vi "Refresh Item.vi"(8 "error in (no error)":errorcluster, 10 "Item Index":i32, 11 "BetterBoxHandle in":refnum<class "BetterBoxHandle.lvclass">) -> (0 "error out":errorcluster, 3 "BetterBoxHandle out":refnum<class "BetterBoxHandle.lvclass">)   [LabVIEW 2020, in "BetterDragAndDrop.lvlib" / "BetterBoxHandle.lvclass"]
uses:
  BetterBoxHandle.lvclass
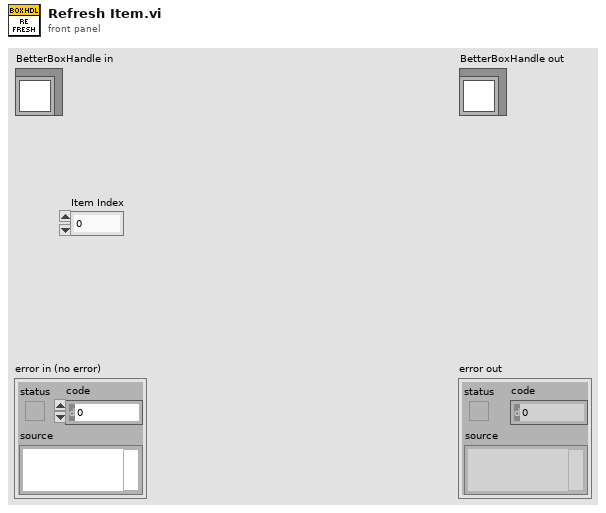
[diagram p1: front panel]
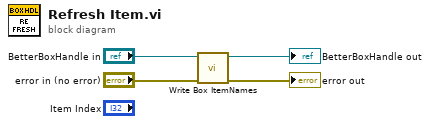
[diagram p0: block diagram]
diagram:
  n1 = call-dynamic "Write Box ItemNames.vi"("error in (no error)"="error in (no error)", "BetterBoxHandle in"="BetterBoxHandle in") -> ("error out"=→"error out":errorcluster, "BetterBoxHandle out"=→"BetterBoxHandle out":refnum<class "BetterBoxHandle.lvclass">)  [unwired: 8 in]
